vi "WPI_CameraIsSimulated.vi"(11 "Camera Address":string) -> (3 "Simulated":bool)   [LabVIEW 2017]
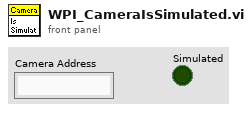
[diagram p1: front panel]
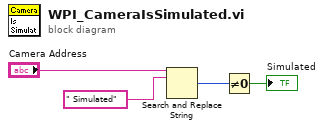
[diagram p0: block diagram]
diagram:
  n1 = Search and Replace String(input string="Camera Address", search string=" Simulated") -> (number of replacements=w2:i32)  [unwired: 6 in, 3 out]
  n2 = Not Equal To 0?(x=w2) -> (x != 0?=→"Simulated":bool)
